vi "SimpleFunctionalTest.vi"() -> (0 "test OK":bool)   [LabVIEW 2014]
panel:
  out "Indicators_list":T1(array[cluster])
  out "Controls_list":T1(array[cluster])
  out "error get":errorcluster
  out "error set":errorcluster
  out "output values":string[](array[string])=["-5", "adios", "false", "0,000000", "10,000000"]
  in  "output variables":string[](array[string])=["intout", "stringout", "booleanout", "doubleout", "time"]
  out "error close":errorcluster
  out "error stop":errorcluster
  out "error start":errorcluster
  out "error open":errorcluster
  in  "input values":string[](array[string])=["-5", "false", "adios", "0,000000"]
  in  "input variables":string[](array[string])=["intin", "booleanin", "stringin", "doublein"]
  in  "Experience ID":string="TestOK"
  # "Simple functional test"
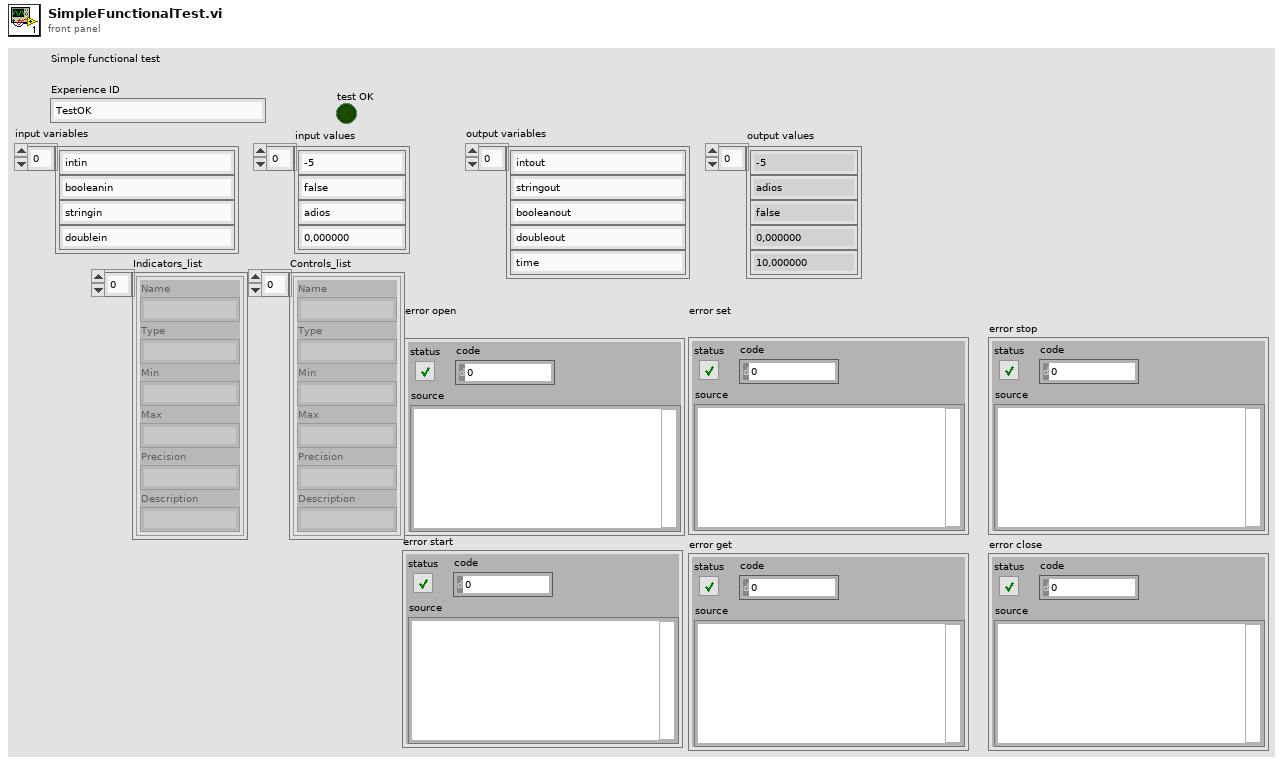
[diagram p1: front panel]
types:
  T1 = cluster{"Name":string, "Type":string, "Min":string, "Max":string, "Precision":string, "Description":string}[]
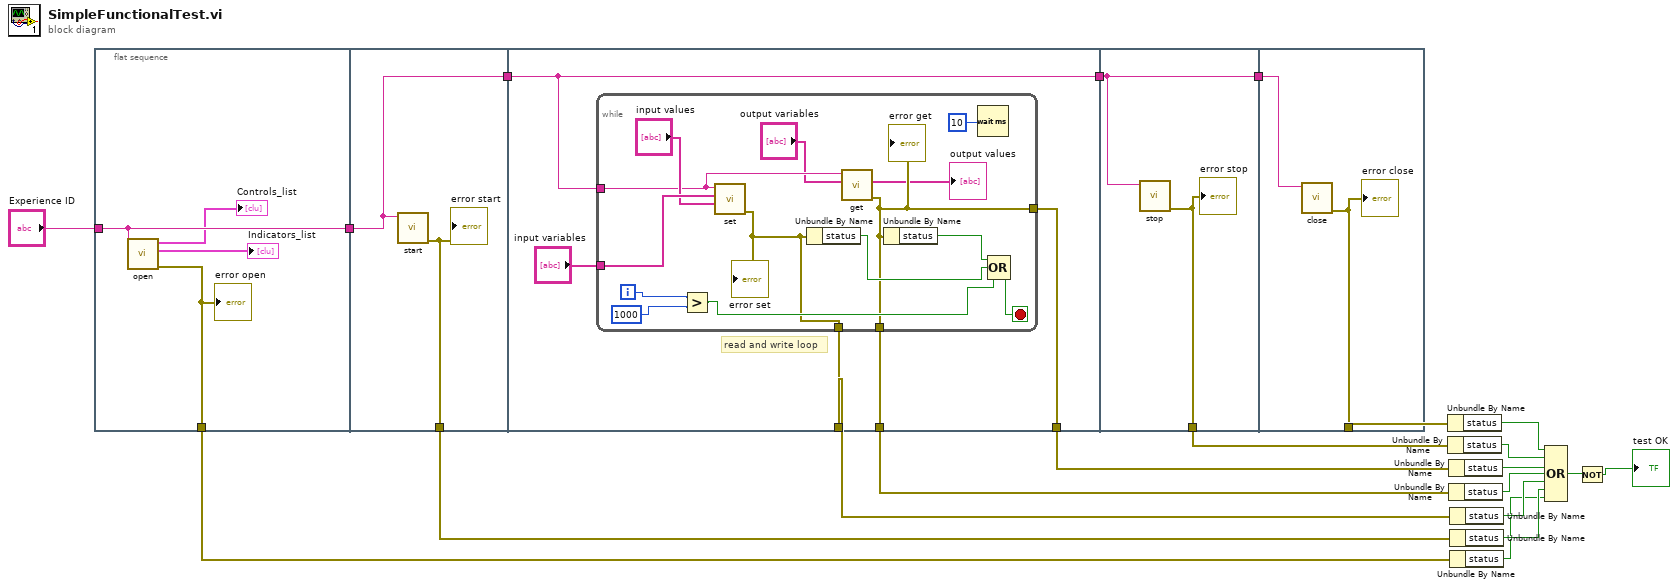
[diagram p0: block diagram]
diagram:
  n1 = flat-sequence {
    tunnel: "Experience ID" -> [w25]
    tunnel: [w25] -> w20
    tunnel: [w24] -> w8
    tunnel: w20 -> [w27]
    tunnel: [w27] -> w19
    tunnel: [w26] -> w9
    tunnel: w19 -> [w32]
    tunnel: [w32] -> w18
    tunnel: [w31] -> w12
    tunnel: [w30] -> w10
    tunnel: [w29] -> w11
    tunnel: w18 -> [w48]
    tunnel: [w48] -> w17
    tunnel: [w47] -> w14
    tunnel: w17 -> [w50]
    tunnel: [w49] -> w15
    frame #0 {
      n2 = call "open.vi"("Experience ID"=w25) -> ("error out"=w24:errorcluster, "Indicators_list"=→"Indicators_list":T1, "Controls_list"=→"Controls_list":T1)  [unwired: 8 in]
      "error open" <- w24
    }
    frame #1 {
      n3 = call "start.vi"("Experience ID"=w27) -> ("error out"=w26:errorcluster)  [unwired: 10 in]
      "error start" <- w26
    }
    frame #2 {
      # "read and write loop"
      n4 = while {
        tunnel: [w36] -> w31
        tunnel: w32 -> [w35]
        tunnel: [w37] -> w30
        tunnel: [w36] -> w29
        tunnel: "input variables" -> [w39]
        i -> [w45]
        stop <- w40 stop-if-true
        n5 = Greater?(x=w45, y=1000) -> (0:w41:bool)
        n6 = call "set.vi"("values"="input values", "variables"=w39, "Experience ID"=w35) -> ("error out"=w37:errorcluster)  [unwired: 8 in]
        "error set" <- w37
        n7 = Unbundle By Name(w37) -> ("status"=w42:bool)
        n8 = call "get.vi"("variables"="output variables", "Experience ID"=w35) -> ("error out"=w36:errorcluster, "values"=→"output values":string[])  [unwired: 7 in, 1 out]
        "error get" <- w36
        n9 = Unbundle By Name(w36) -> ("status"=w43:bool)
        n10 = Wait (ms)(milliseconds to wait=u32 10) -> ()  [unwired: 1 out]
        n11 = Compound Arithmetic op=OR(w43, w42, w41) -> (w40:bool)
      }
    }
    frame #3 {
      n12 = call "stop.vi"("Experience ID"=w48) -> ("error out"=w47:errorcluster)  [unwired: 10 in]
      "error stop" <- w47
    }
    frame #4 {
      n13 = call "close.vi"("Experience ID"=w50) -> ("error out"=w49:errorcluster)  [unwired: 10 in]
      "error close" <- w49
    }
  }
  n14 = Unbundle By Name(w15) -> ("status"=w16:bool)
  n15 = Unbundle By Name(w14) -> ("status"=w13:bool)
  n16 = Unbundle By Name(w12) -> ("status"=w7:bool)
  n17 = Unbundle By Name(w11) -> ("status"=w6:bool)
  n18 = Unbundle By Name(w10) -> ("status"=w5:bool)
  n19 = Unbundle By Name(w9) -> ("status"=w4:bool)
  n20 = Unbundle By Name(w8) -> ("status"=w3:bool)
  n21 = Compound Arithmetic op=OR(w16, w13, w7, w6, w5, w4, w3) -> (w2:bool)
  n22 = Not(x=w2) -> (.not. x?=→"test OK":bool)
